vi "niRFUtil WFM Correlate (real wfm).vi"(1 "Reference Waveform":T1 {"y" min=0 max=127 format="%.2f"; "dx" format="%^.2e"; "x0" format="%^.2e"}, 2 "Waveform In":T1 {"y" min=0 max=127 format="%.2f"; "dx" format="%^.2e"; "x0" format="%^.2e"}) -> (0 "Waveform Out":T1 {"y" min=0 max=127 format="%.2f"; "dx" format="%^.2e"; "x0" format="%^.2e"})   [LabVIEW 2015, in "niRFUtil.lvlib"]
doc: "(c) Copyright 2006, National Instruments, Inc. This VI may not be duplicated, sold, or distributed without written consent from National Instruments."
uses:
  niRFUtil.lvlib
  Includes/niRFUtil INC Real Waveform.ctl
  Includes/niRFUtil INC Real Array.ctl
  <vilib>/Analysis/2dsp.llb/1D Cross Correlation (DBL).vi
  <vilib>/Analysis/NI_AALPro.lvlib
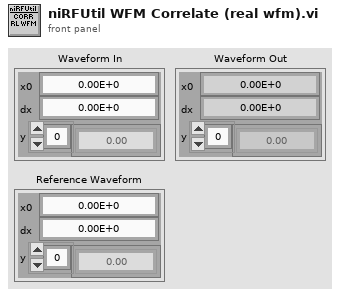
[diagram p1: front panel]
types:
  T1 = typedef "niRFUtil.lvlib/niRFUtil INC Real Waveform.ctl" = cluster{"x0":dbl, "dx":dbl, "y":T2}
  T2 = typedef "niRFUtil.lvlib/niRFUtil INC Real Array.ctl" = sgl[]
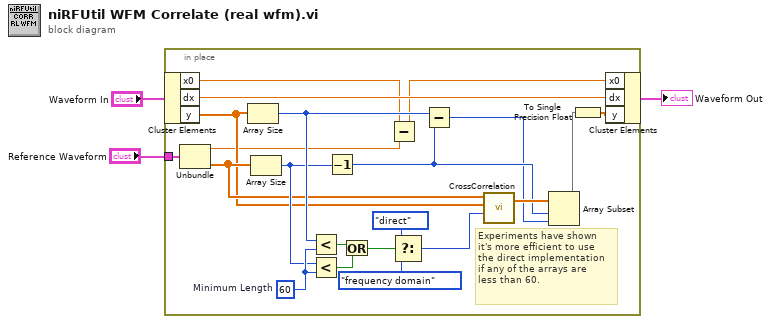
[diagram p0: block diagram]
diagram:
  n1 = in-place {
    in-place-border: "Reference Waveform" -> [w11]
    w23 = 60  # Minimum Length
    # "Experiments have shown\nit's more efficient to use\nthe direct implementation\nif any of the arrays are\nless than 60."
    n2 = in-place-cluster #1("Waveform In") -> ("x0"=w5:dbl, "dx"=w16:dbl, "y"=w7:T2)
    n3 = Unbundle(w11) -> ("x0"=w6:dbl, "y"=w8:T2)  [unwired: 1 out]
    n4 = Array Size(array=w7) -> (size(s)=w13:i32)
    n5 = Array Size(array=w8) -> (size(s)=w12:i32)
    n6 = Less?(x=w13, y=w23) -> (x < y?=w22:bool)
    n7 = Less?(x=w12, y=w23) -> (x < y?=w21:bool)
    n8 = Decrement(x=w12) -> (x-1=w15:i32)
    n9 = Or(x=w22, y=w21) -> (x .or. y?=w20:bool)
    n10 = Subtract(x=w5, y=w6) -> (x-y=w4:dbl)
    n11 = Select(t=enum32{"direct", "frequency domain"}."direct" ("algorithm"), s=w20, f=enum32{"direct", "frequency domain"}."frequency domain" ("algorithm")) -> (s? t:f=w17:enum32{"direct", "frequency domain"})
    n12 = Subtract(x=w13, y=w15) -> (x-y=w14:i32)
    n13 = call-poly <vilib>:"CrossCorrelation.vi"("algorithm"=w17, "Y"=w7, "X"=w8) -> ("Rxy"=w24:dbl[])  [unwired: 7 in, 1 out]
    n14 = Array Subset(array=w24, index=w15, length=w14) -> (w10:dbl[])
    n15 = To Single Precision Float(number=w10) -> (single precision float=w9:sgl[])
    n16 = in-place-cluster #1("x0"=w4, "dx"=w16, "y"=w9) -> (→"Waveform Out":T1)
  }
